vi "Measurements Graph_V2_Cpd.vi"(0 "Bias Voltage":dbl[](array[numeric]), 2 "Stop_V":dbl, 5 "Resitance":dbl[](array[numeric]), 7 "Cpd":dbl[](array[numeric]), 11 "Error In":errorcluster) -> (4 "Graph Cluster":T1, 15 "Error Out":errorcluster)   [LabVIEW 2013]
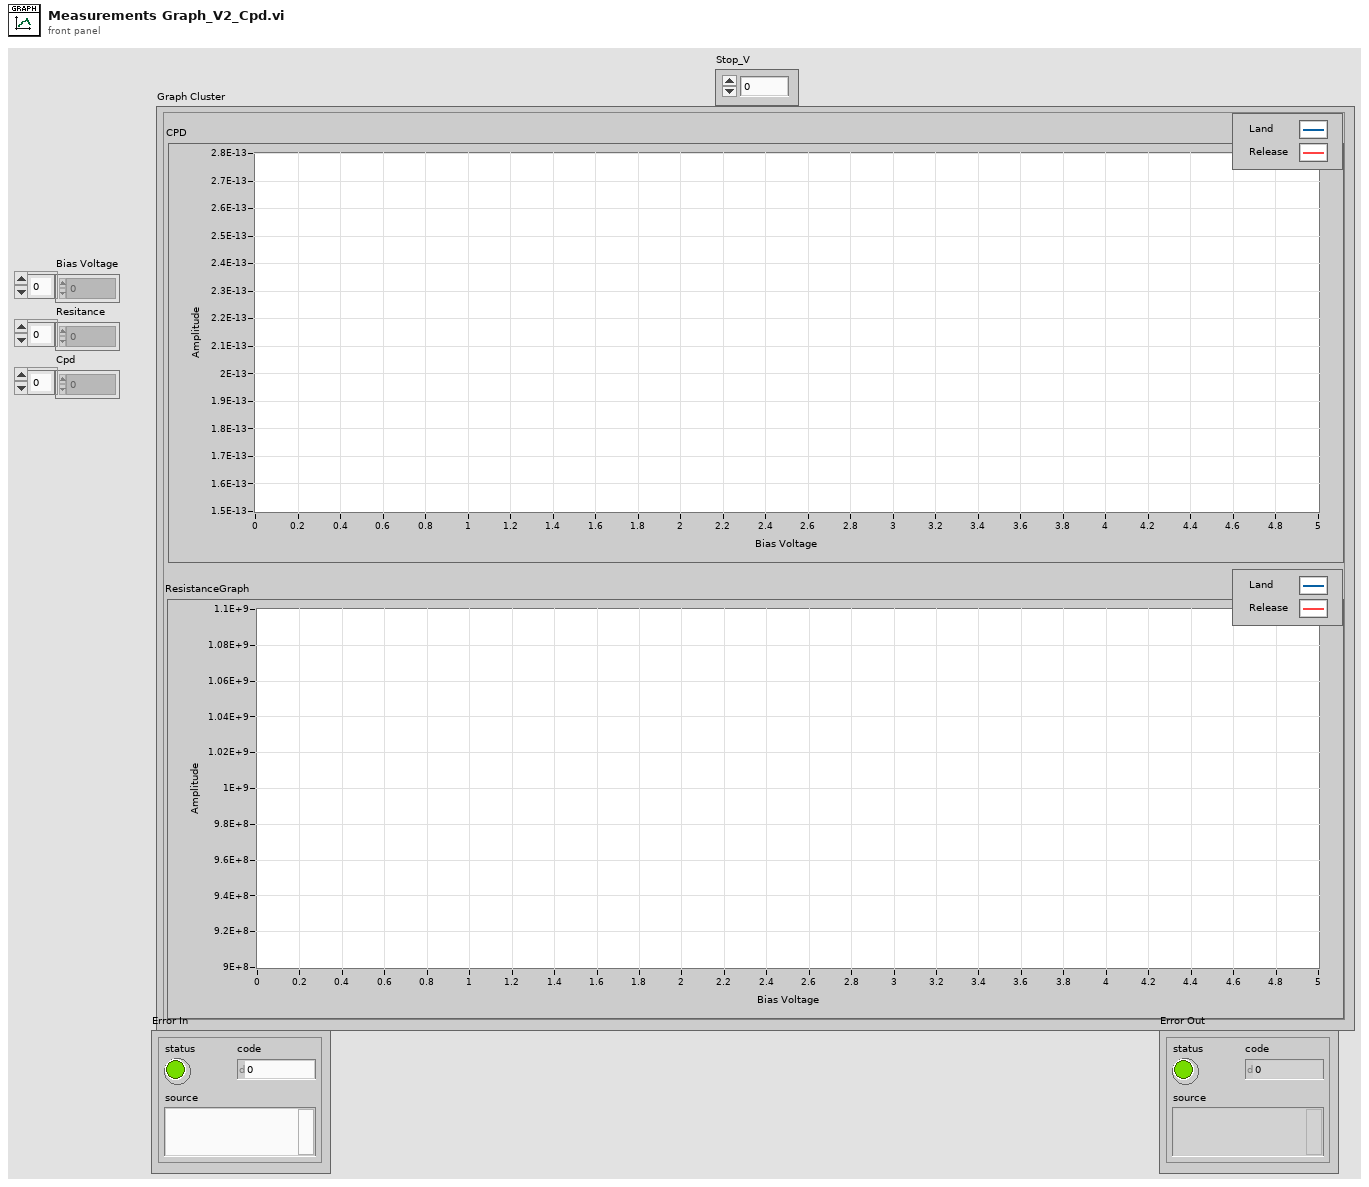
[diagram p1: front panel]
types:
  T1 = cluster{"ResistanceGraph":cluster{dbl[], dbl[]}[], "CPD":cluster{dbl[], dbl[]}[]}
  T2 = cluster{cluster{dbl[], dbl[]}[], cluster{dbl[], dbl[]}[]}
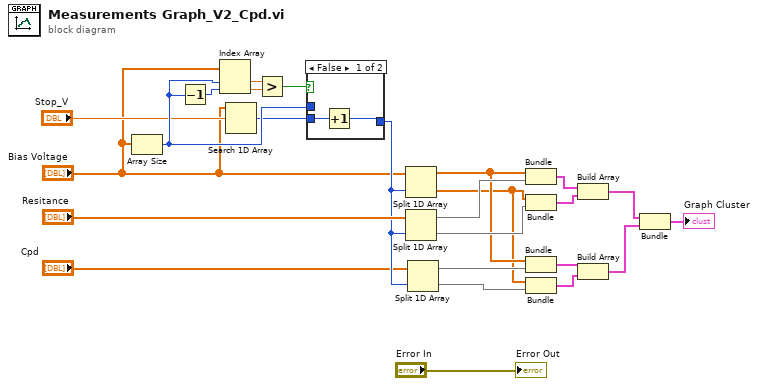
[diagram p0: block diagram]
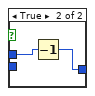
[diagram p2: hidden frame]
diagram:
  n1 = Array Size(array="Bias Voltage") -> (size(s)=w8:i32)
  n2 = Decrement(x=w8) -> (x-1=w11:i32)
  n3 = Index Array(array="Bias Voltage", index #1=w8, index #2=w11) -> (element #1=w9:dbl, element #2=w10:dbl)
  n4 = Search 1D Array(1D array="Bias Voltage", element="Stop_V") -> (index of element=w4:i32)  [unwired: 1 in]
  n5 = Greater?(x=w9, y=w10) -> (0:w3:bool)
  n6 = case shown="False" w3 {
    tunnel: w8 -> [_ w29]
    tunnel: [w26 w28] -> w7
    tunnel: w4 -> [w27 _]
    frame False {
      n7 = Increment(x=w27) -> (x+1=w26:i32)
    }
    frame True {
      n8 = Decrement(x=w29) -> (x-1=w28:i32)
    }
  }
  n9 = Split 1D Array(array="Bias Voltage", index=w7) -> (first subarray=w16:dbl[], second subarray=w15:dbl[])
  n10 = Split 1D Array(array="Resitance", index=w7) -> (first subarray=w24:dbl[], second subarray=w23:dbl[])
  n11 = Split 1D Array(array="Cpd", index=w7) -> (first subarray=w18:dbl[], second subarray=w17:dbl[])
  n12 = Bundle(w16, w24) -> (w22:cluster{dbl[], dbl[]})  [unwired: 1 in]
  n13 = Bundle(w15, w23) -> (w21:cluster{dbl[], dbl[]})  [unwired: 1 in]
  n14 = Bundle(w16, w18) -> (w20:cluster{dbl[], dbl[]})  [unwired: 1 in]
  n15 = Bundle(w15, w17) -> (w19:cluster{dbl[], dbl[]})  [unwired: 1 in]
  n16 = Build Array(w22, w21) -> (w14:cluster{dbl[], dbl[]}[])
  n17 = Build Array(w20, w19) -> (w13:cluster{dbl[], dbl[]}[])
  n18 = Bundle(w14, w13) -> (→"Graph Cluster":T2)  [unwired: 1 in]
  "Error Out" <- "Error In"
